vi "Get Service Descriptor.vi"(8 "error in":errorcluster) -> (0 "error out":errorcluster, 3 "service descriptor":T1)   [LabVIEW 2021, in "DAQmxMeasurement1.lvlib"]
uses:
  DAQmxMeasurement1.lvlib
  <vilib>/Plug-In SDKs/Measurements/Helpers/TypeDefs/Service Descriptor.ctl
  <vilib>/Plug-In SDKs/Measurements/Helpers/TypeDefs/Measurement Details.ctl
  <vilib>/Plug-In SDKs/Measurements/Helpers/TypeDefs/Measurement Annotation.ctl
  <vilib>/Plug-In SDKs/Measurements/NI Measurement Plug-In SDK.lvlib
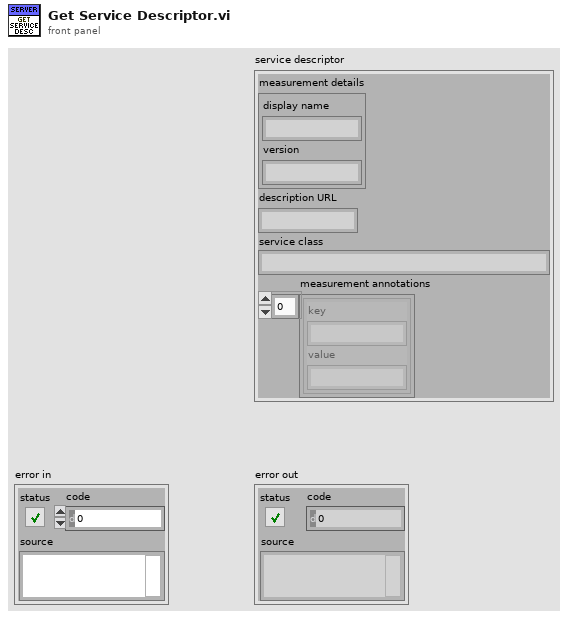
[diagram p1: front panel]
types:
  T1 = typedef "NI Measurement Plug-In SDK.lvlib/Service Descriptor.ctl" = cluster{"measurement details":T2, "description URL":string, "service class":string, "measurement annotations":T3[]}
  T2 = typedef "NI Measurement Plug-In SDK.lvlib/Measurement Details.ctl" = cluster{"display name":string, "version":string}
  T3 = typedef "NI Measurement Plug-In SDK.lvlib/Measurement Annotation.ctl" = cluster{"key":string, "value":string}
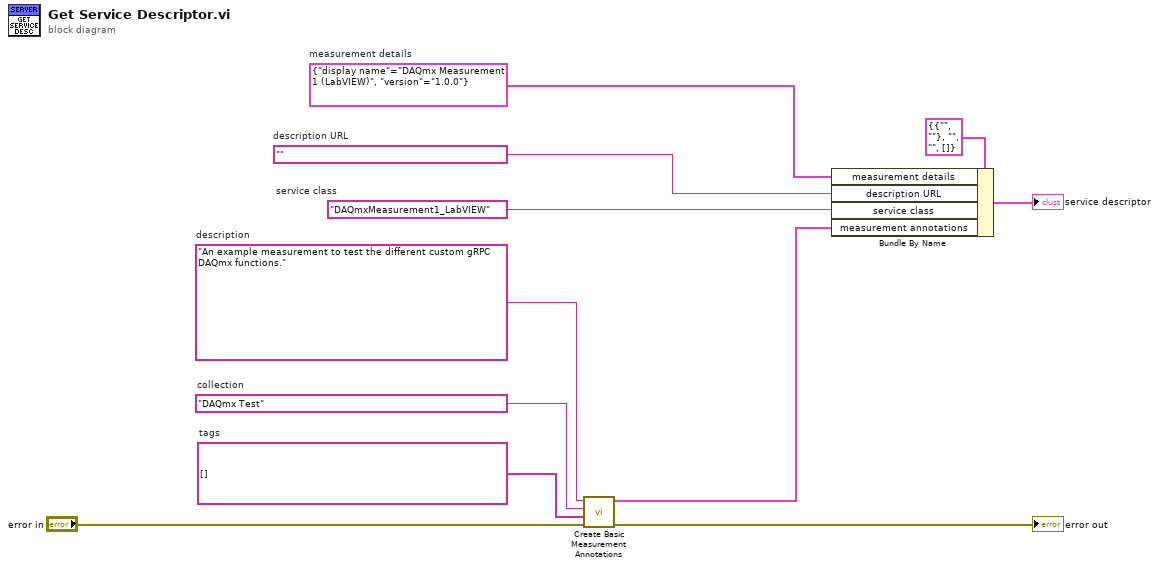
[diagram p0: block diagram]
diagram:
  w5 = ""  # description URL
  w7 = string[] []  # tags
  w8 = "DAQmx Test"  # collection
  w9 = "An example measurement to test the different custom gRPC DAQmx functions."  # description
  w6 = T2 {"display name"="DAQmx Measurement 1 (LabVIEW)", "version"="1.0.0"}  # measurement details
  w4 = "DAQmxMeasurement1_LabVIEW"  # service class
  n1 = call <vilib>:"Create Basic Measurement Annotations.vi"("error in"="error in", "tags"=w7, "collection"=w8, "description"=w9) -> ("error out"=→"error out":errorcluster, "measurement annotations"=w3:T3[])  [unwired: 6 in]
  n2 = Bundle By Name(cluster=T1 {"measurement details"={"display name"="", "version"=""}, "description URL"="", "service class"="", "measurement annotations"=[]} ("service descriptor"), "measurement details"=w6, "description URL"=w5, "service class"=w4, "measurement annotations"=w3) -> (→"service descriptor":T1)
